vi "Signal Generator.vi"(7 "Sample Frequency":dbl=1000000.0, 8 "error in (no error)":errorcluster, 9 "#Samples":dbl=1000.0, 10 "frequency":dbl=1000.0 format="%.2p", 11 "Signal Type":enum16{"Sine", "Square", "Triangle", "Sawtooth"}(ring)) -> (0 "error out":errorcluster, 3 "Data":dbl[](array[numeric]))   [LabVIEW 2010]
uses:
  <vilib>/measure/NI_MABase.lvlib
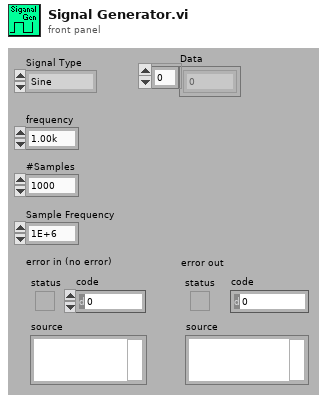
[diagram p1: front panel]
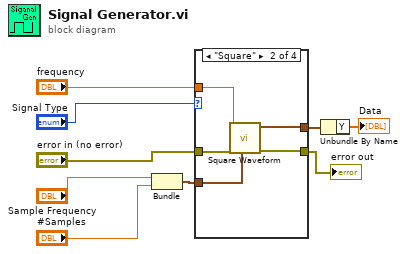
[diagram p0: block diagram]
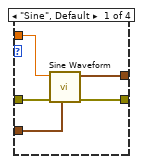
[diagram p2: hidden frame]
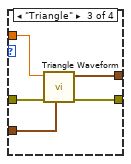
[diagram p3: hidden frame]
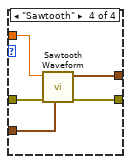
[diagram p4: hidden frame]
diagram:
  n1 = Bundle("Sample Frequency"="Sample Frequency", "#Samples"="#Samples") -> (w3:cluster{"Sample Frequency":dbl, "#Samples":dbl})  [unwired: 1 in]
  n2 = case shown="\"Square\"" "Signal Type" {
    tunnel: [w14 w19 w24 w29] -> w9
    tunnel: "frequency" -> [w13 w18 w23 w28]
    tunnel: w3 -> [w12 w17 w22 w27]
    tunnel: "error in (no error)" -> [w10 w16 w21 w26]
    tunnel: [w11 w15 w20 w25] -> w1
    frame "Sine", Default {
      n3 = call <vilib>:"Sine Waveform.vi"("sampling info"=w12, "error in (no error)"=w10, "frequency"=w13) -> ("error out"=w11:errorcluster, "signal out"=w14:waveform(dbl))  [unwired: 7 in]
    }
    frame "Square" {
      n4 = call <vilib>:"Square Waveform.vi"("sampling info"=w17, "error in (no error)"=w16, "frequency"=w18) -> ("error out"=w15:errorcluster, "signal out"=w19:waveform(dbl))  [unwired: 7 in]
    }
    frame "Triangle" {
      n5 = call <vilib>:"Triangle Waveform.vi"("sampling info"=w22, "error in (no error)"=w21, "frequency"=w23) -> ("error out"=w20:errorcluster, "signal out"=w24:waveform(dbl))  [unwired: 7 in]
    }
    frame "Sawtooth" {
      n6 = call <vilib>:"Sawtooth Waveform.vi"("sampling info"=w27, "error in (no error)"=w26, "frequency"=w28) -> ("error out"=w25:errorcluster, "signal out"=w29:waveform(dbl))  [unwired: 7 in]
    }
  }
  "error out" <- w1
  n7 = Unbundle By Name(w9) -> ("Y"=→"Data":dbl[])
